vi "Change_Pelletron_Status.vi"(8 "error in (no error)":errorcluster, 9 "Write Value":dbl, 10 "Write Selector":u16(ring) items=["GV", "Blower", "Main Power Supply", "Chain Power Supply", "Chain", "Rotating Shaft", "Power Supply Voltage", "Control Mode", "Control Mode Reference", "Chain Bypass", "Rotating Shaft Bypass", "Spark Counter", "Spark Limit", "Threshold", "Spark Counter Reset", "Ion Filament"], 11 "AccelNET.lvlib:TCP.lvclass":refnum<class "TCP.lvclass">) -> (0 "error out":errorcluster)   [LabVIEW 2012, in "AccelNET.lvlib" / "TCP.lvclass"]
uses:
  TCP.lvclass
  TCP.lvclass/TCP.ctl
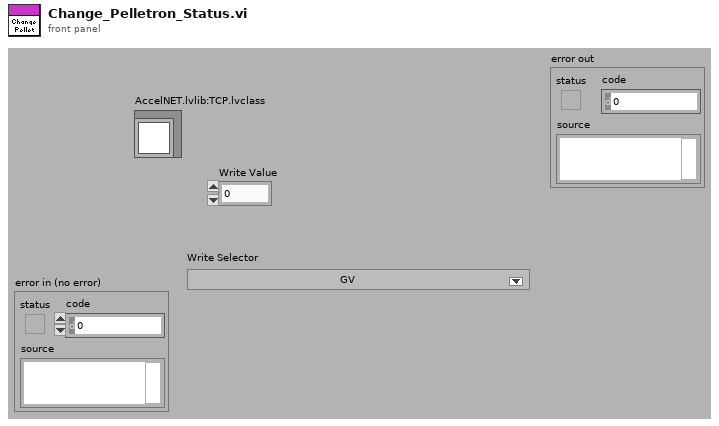
[diagram p1: front panel]
types:
  T1 = enum16{"Standard", "Buffered", "CRLF", "Immediate"}
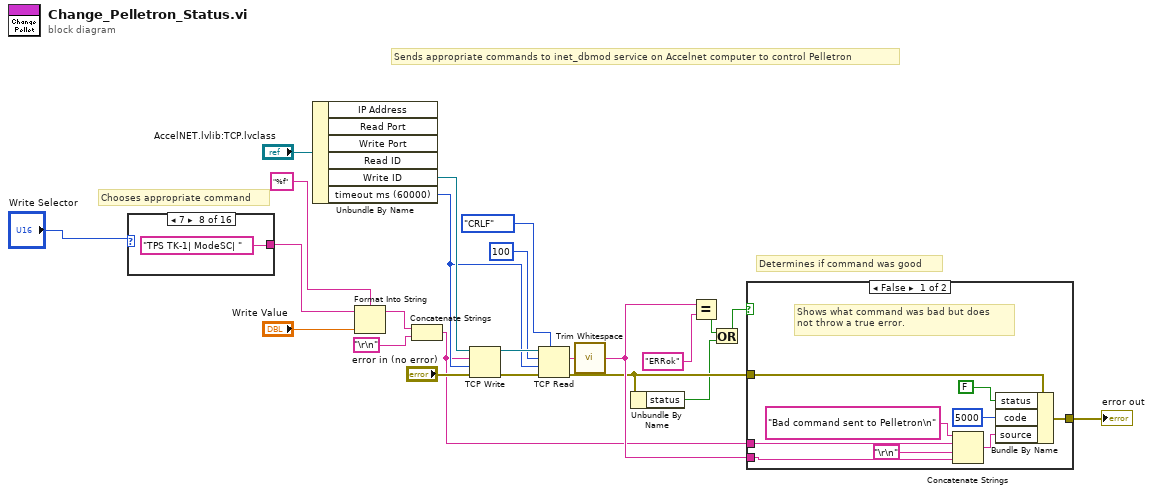
[diagram p0: block diagram]
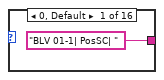
[diagram p3: hidden frame]
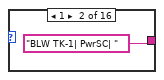
[diagram p4: hidden frame]
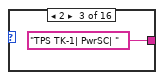
[diagram p5: hidden frame]
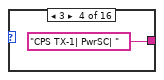
[diagram p6: hidden frame]
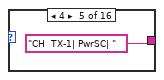
[diagram p7: hidden frame]
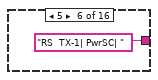
[diagram p8: hidden frame]
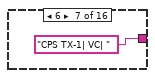
[diagram p9: hidden frame]
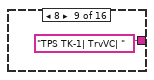
[diagram p10: hidden frame]
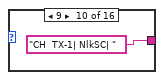
[diagram p11: hidden frame]
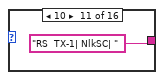
[diagram p12: hidden frame]
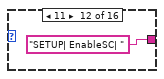
[diagram p13: hidden frame]
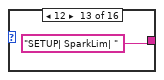
[diagram p14: hidden frame]
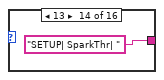
[diagram p15: hidden frame]
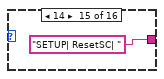
[diagram p16: hidden frame]
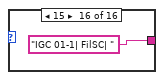
[diagram p17: hidden frame]
diagram:
  # "Determines if command was good"
  # "Chooses appropriate command"
  # "Sends appropriate commands to inet_dbmod service on Accelnet computer to control Pelletron"
  n1 = case shown="7" "Write Selector" {
    tunnel: ["BLV 01-1| PosSC| " "BLW TK-1| PwrSC| " "TPS TK-1| PwrSC| " "CPS TX-1| PwrSC| " "CH  TX-1| PwrSC| " "RS  TX-1| PwrSC| " "CPS TX-1| VC| " "TPS TK-1| ModeSC| " "TPS TK-1| TrvVC| " "CH  TX-1| NlkSC| " "RS  TX-1| NlkSC| " "SETUP| EnableSC| " "SETUP| SparkLim| " "SETUP| SparkThr| " "SETUP| ResetSC| " "IGC 01-1| FilSC| "] -> w19
    frame 0, Default {
    }
    frame 1 {
    }
    frame 2 {
    }
    frame 3 {
    }
    frame 4 {
    }
    frame 5 {
    }
    frame 6 {
    }
    frame 7 {
    }
    frame 8 {
    }
    frame 9 {
    }
    frame 10 {
    }
    frame 11 {
    }
    frame 12 {
    }
    frame 13 {
    }
    frame 14 {
    }
    frame 15 {
    }
  }
  n2 = Unbundle By Name("AccelNET.lvlib:TCP.lvclass") -> ("Write ID"=w22:refnum<k5>, "timeout ms (60000)"=w15:i32)  [unwired: 4 out]
  n3 = Format Into String(format string="%f", initial string=w19, "Write Value") -> (resulting string=w11:string)  [unwired: 1 in, 1 out]
  n4 = Concatenate Strings(w11, "\r\n") -> (w2:string)
  n5 = TCP Write(connection ID=w22, data in=w2, error in (no error)="error in (no error)", 9:w15) -> (connection ID out=w17:refnum<k5>, error out=w14:errorcluster)  [unwired: 1 out]
  n6 = TCP Read(connection ID=w17, bytes to read=100, error in (no error)=w14, 7:T1."CRLF" ("mode (standard)"), 9:w15) -> (data out=w8:string, error out=w6:errorcluster)  [unwired: 1 out]
  n7 = call <vilib>:"Trim Whitespace.vi"("string"=w8) -> ("trimmed string"=w7:string)  [unwired: 1 in]
  n8 = Unbundle By Name(w6) -> ("status"=w4:bool)
  n9 = Equal?(x=w7, y="ERRok") -> (x = y?=w5:bool)
  n10 = Or(x=w5, y=w4) -> (x .or. y?=w3:bool)
  n11 = case shown="False" w3 {
    tunnel: w6 -> [w48 w49]
    tunnel: [w46 w49] -> w10
    tunnel: w2 -> [w43 _]
    tunnel: w7 -> [w41 _]
    frame False {
      # "Shows what command was bad but does\nnot throw a true error."
      n12 = Concatenate Strings("Bad command sent to Pelletron\n" ("source"), w43, "\r\n", w41) -> (w42:string)
      n13 = Bundle By Name(cluster=w48, "status"=FALSE, "code"=5000, "source"=w42) -> (w46:errorcluster)
    }
    frame True {
    }
  }
  "error out" <- w10
